vi "QuadBot SetAllAngles.vi"(8 "error in (no error)":errorcluster, 9 "Speed":u32, 10 "angles":dbl[](array[numeric]), 11 "Cluster":cluster{"Ctl Refnum":refnum<vi>}) -> (0 "error out":errorcluster, 2 "Ok?":bool, 3 "Cluster 2":cluster{"Ctl Refnum 2":refnum<vi>})   [LabVIEW 2015]
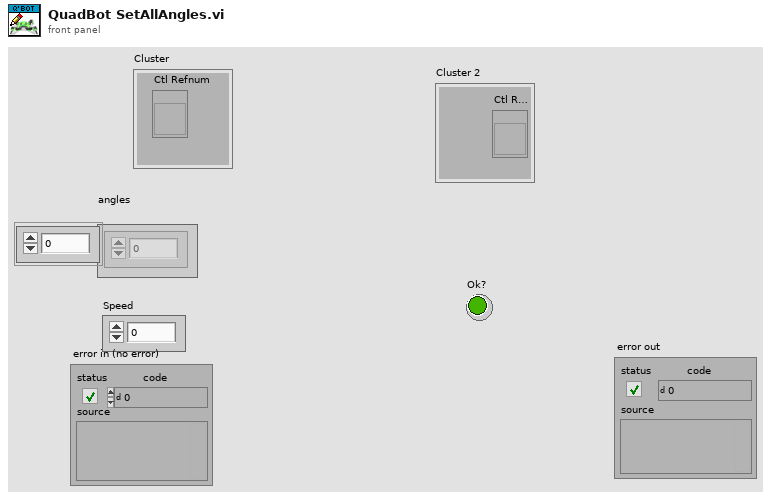
[diagram p1: front panel]
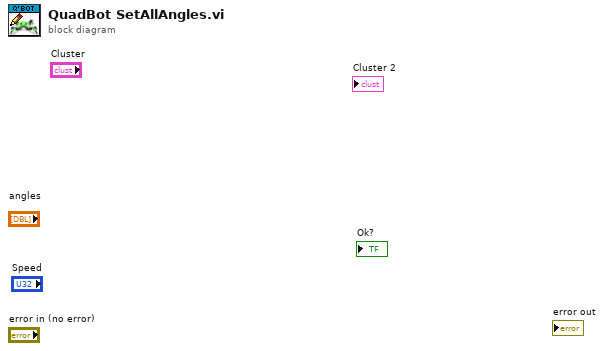
[diagram p0: block diagram]
diagram:
